vi "Display_blocks.vi"(6 "Block No":i32, 10 "Block average display":cluster{"Name":string, "Include":bool}[](array[cluster])) -> (0 "u^4":dbl[][](graph), 1 "u^3":dbl[][](graph), 2 "uv":dbl[][](graph), 3 "u^2":dbl[][](graph), 4 "U":dbl[][](graph))   [LabVIEW 2011]
uses:
  Globals/Meas_global.vi
panel:
  in  "3D Cross":dbl[][][](array[numeric]) format="%.2f"
  in  "3D single":dbl[][][](array[numeric]) format="%.2f"
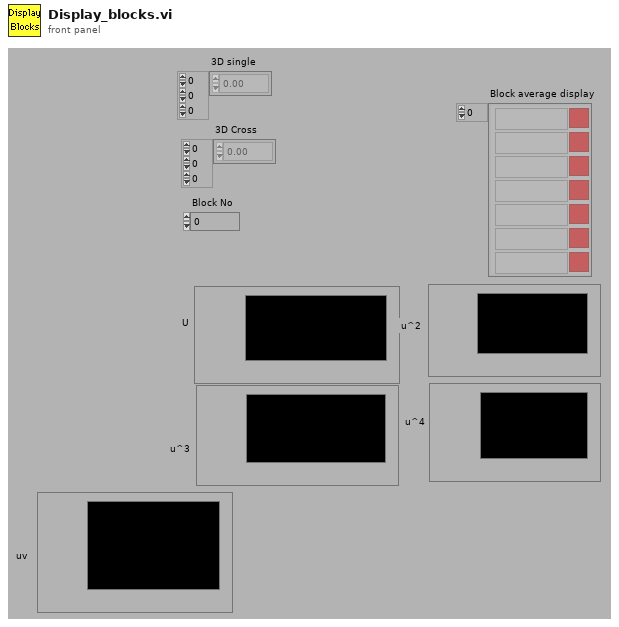
[diagram p1: front panel]
types:
  T1 = typedef "Analysis_info_cluster.ctl" = cluster{"Colour":u32, "Inst type":T2, "Inst name":string, "Symbol":string, "Code name":string, "Extra Info":string, "Inst Array":T3, "Index":i32, "Voltage Index":i32, "Extra Titles":string[], "Extra Values":string[], "Eng Values":dbl[], "Time (ms)":dbl[], "TT / Voltage":dbl[], "U":dbl, "u^2":dbl, "u^3":dbl, "u^4":dbl, "Skew_u":dbl, "Kurt_u":dbl, "Sd Error in Mean":dbl, "% u'/U":dbl, "X":dbl, "Y":dbl, "Z":dbl, "Spectra":T4, "Autocorrelation":T4, "Timescale integral to 25%":dbl, "Sd Error in Variance":dbl, "Calib File":path, "Calib Constants":dbl[], "Histogram":T4, "Output Position":bool, "Full Stats":bool}
  T2 = typedef "Inst_type.ctl" = enum16{"Propeller anemometer", "Raw voltage", "Pressure Transducer", "Pitot-static tube", "Preston tube", "Hot wire", "Cross wire 1", "Cross wire 2", "Generic Linear", "Generic Polynomial", "Generic BackPoly", "Fast FID", "Thermocouple", "Cold wire", "Pulsed Wire", "LDA Vel", "LDA Tran time", "LDA Arr time"}
  T3 = typedef "Instrument_Array.ctl" = enum16{"PWA", "LDA", "Analogue"}
  T4 = typedef "XY_Plot_Cluster.ctl" = cluster{"First Name":string, "Second Name":string, "X axis name":string, "Y axis name":string, "X array":dbl[], "Y array":dbl[]}
  T5 = typedef "Correlation_cluster1.ctl" = cluster{"U inst":string, "uw":dbl, "u^2w":dbl, "uw^2":dbl, "uw/u'w'":dbl, "W inst":string, "uw^3":dbl, "u^3w":dbl, "u^2w^2":dbl, "Index U":i32, "Index W":i32}
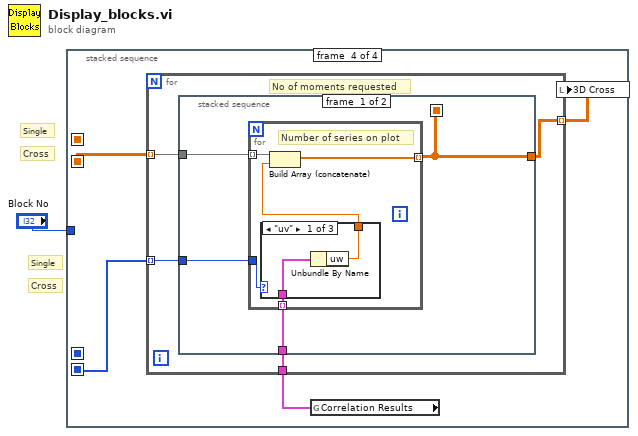
[diagram p0: block diagram]
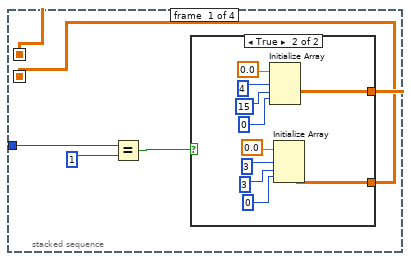
[diagram p2: hidden frame]
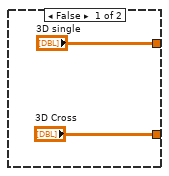
[diagram p3: hidden frame]
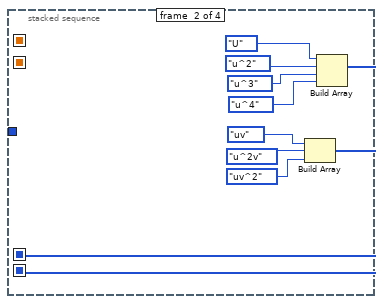
[diagram p4: hidden frame]
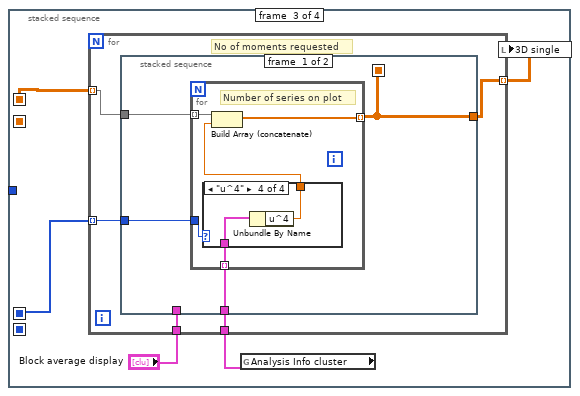
[diagram p5: hidden frame]
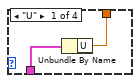
[diagram p6: hidden frame]
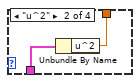
[diagram p7: hidden frame]
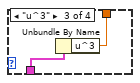
[diagram p8: hidden frame]
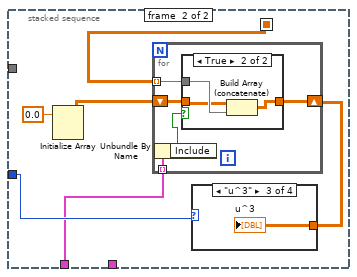
[diagram p9: hidden frame]
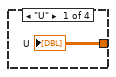
[diagram p10: hidden frame]
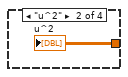
[diagram p11: hidden frame]
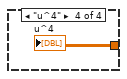
[diagram p12: hidden frame]
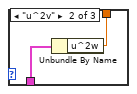
[diagram p14: hidden frame]
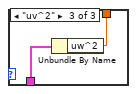
[diagram p15: hidden frame]
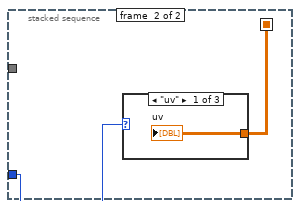
[diagram p16: hidden frame]
diagram:
  # "Single"
  # "Cross"
  # "Cross"
  # "Single"
  n1 = stacked-sequence {
    seq-local: [_ w27 _ _] -> [_ _ w32 _]
    seq-local: [_ w26 _ _] -> [_ _ _ w75]
    seq-local: [w4 _ _ _] -> [_ _ w31 _]
    seq-local: [w3 _ _ _] -> [_ _ _ w76]
    tunnel: "Block No" -> [w2 _ _ _]
    frame #0 {
      n2 = Equal?(x=w2, y=1) -> (x = y?=w5:bool)
      n3 = case shown="True" w5 {
        tunnel: ["3D single" w14] -> w4
        tunnel: ["3D Cross" w9] -> w3
        frame False {
        }
        frame True {
          n4 = Initialize Array(0.0, 4, 15, 0) -> (w14:dbl[][][])
          n5 = Initialize Array(0.0, 3, 3, 0) -> (w9:dbl[][][])
        }
      }
    }
    frame #1 {
      n6 = Build Array(enum16{"uv", "u^2v", "uv^2"}."uv", enum16{"uv", "u^2v", "uv^2"}."u^2v", enum16{"uv", "u^2v", "uv^2"}."uv^2") -> (w26:enum16{"uv", "u^2v", "uv^2"}[])
      n7 = Build Array(enum16{"U", "u^2", "u^3", "u^4"}."U", enum16{"U", "u^2", "u^3", "u^4"}."u^2", enum16{"U", "u^2", "u^3", "u^4"}."u^3", enum16{"U", "u^2", "u^3", "u^4"}."u^4") -> (w27:enum16{"U", "u^2", "u^3", "u^4"}[])
    }
    frame #2 {
      n8 = global read "Meas_global.vi" "Analysis Info cluster"() -> (w28:T1[])
      n9 = for {
        tunnel: w31 -> [w37] mode=indexing
        tunnel: w32 -> [w36] mode=indexing
        tunnel: [w35] -> w30 mode=indexing
        tunnel: w28 -> [w34]
        tunnel: "Block average display" -> [w33]
        # "No of moments requested"
        n10 = stacked-sequence {
          seq-local: [w39 _] -> [_ w59]
          tunnel: [w39 _] -> w35
          tunnel: w36 -> [w41 w57]
          tunnel: w37 -> [w40 _]
          tunnel: w34 -> [w38 _]
          tunnel: w33 -> [_ w55]
          frame #0 {
            n11 = for {
              tunnel: w40 -> [w46] mode=indexing
              tunnel: [w44] -> w39 mode=indexing
              tunnel: w41 -> [w45]
              tunnel: w38 -> [w43] mode=indexing
              # "Number of series on plot"
              n12 = case shown="\"u^4\"" w45 {
                tunnel: [w48 w50 w52 w54] -> w42
                tunnel: w43 -> [w47 w49 w51 w53]
                frame "U" {
                  n13 = Unbundle By Name(w47) -> ("U"=w48:dbl)
                }
                frame "u^2" {
                  n14 = Unbundle By Name(w49) -> ("u^2"=w50:dbl)
                }
                frame "u^3" {
                  n15 = Unbundle By Name(w51) -> ("u^3"=w52:dbl)
                }
                frame "u^4" {
                  n16 = Unbundle By Name(w53) -> ("u^4"=w54:dbl)
                }
              }
              n17 = Build Array (concatenate)(w46, w42) -> (w44:dbl[])
            }
          }
          frame #1 {
            n18 = Initialize Array(0.0) -> (w58:dbl[][])  [unwired: 2 out]
            n19 = for {
              shift-right: [w66] -> w56
              shift-left: w58 -> [w68]
              tunnel: w59 -> [w67] mode=indexing
              tunnel: w55 -> [w65] mode=indexing
              n20 = Unbundle By Name(w65) -> ("Include"=w69:bool)
              n21 = case shown="True" w69 {
                tunnel: [w70 w73] -> w66
                tunnel: w68 -> [w70 w71]
                tunnel: w67 -> [_ w72]
                frame False {
                }
                frame True {
                  n22 = Build Array (concatenate)(w71, w72) -> (w73:dbl[][])
                }
              }
            }
            n23 = case shown="\"u^3\"" w57 {
              tunnel: w56 -> [w61 w62 w63 w64]
              frame "U" {
                "U" <- w61
              }
              frame "u^2" {
                "u^2" <- w62
              }
              frame "u^3" {
                "u^3" <- w63
              }
              frame "u^4" {
                "u^4" <- w64
              }
            }
          }
        }
      }
      n24 = local write "3D single"(w30) -> ()
    }
    frame #3 {
      n25 = global read "Meas_global.vi" "Correlation Results"() -> (w74:T5[])
      n26 = for {
        tunnel: w76 -> [w81] mode=indexing
        tunnel: w75 -> [w80] mode=indexing
        tunnel: [w79] -> w77 mode=indexing
        tunnel: w74 -> [w78]
        # "No of moments requested"
        n27 = stacked-sequence {
          seq-local: [w83 _] -> [_ w97]
          tunnel: [w83 _] -> w79
          tunnel: w80 -> [w85 w98]
          tunnel: w81 -> [w84 _]
          tunnel: w78 -> [w82 _]
          frame #0 {
            n28 = for {
              tunnel: w84 -> [w90] mode=indexing
              tunnel: [w88] -> w83 mode=indexing
              tunnel: w85 -> [w89]
              tunnel: w82 -> [w86] mode=indexing
              # "Number of series on plot"
              n29 = case shown="\"uv\"" w89 {
                tunnel: [w92 w94 w96] -> w87
                tunnel: w86 -> [w91 w93 w95]
                frame "uv" {
                  n30 = Unbundle By Name(w91) -> ("uw"=w92:dbl)
                }
                frame "u^2v" {
                  n31 = Unbundle By Name(w93) -> ("u^2w"=w94:dbl)
                }
                frame "uv^2" {
                  n32 = Unbundle By Name(w95) -> ("uw^2"=w96:dbl)
                }
              }
              n33 = Build Array (concatenate)(w90, w87) -> (w88:dbl[])
            }
          }
          frame #1 {
            n34 = case shown="\"uv\"" w98 {
              tunnel: w97 -> [w99 _ _]
              frame "uv" {
                "uv" <- w99
              }
              frame "u^2v" {
              }
              frame "uv^2" {
              }
            }
          }
        }
      }
      n35 = local write "3D Cross"(w77) -> ()
    }
  }
